vi "Normalize Score.vi"(10 "Value":dbl) -> (2 "Score":dbl)   [LabVIEW 2025]
doc: "Given a value with an ideal value of 1.0, normalize and map to a score that ranges between 0 and 100."
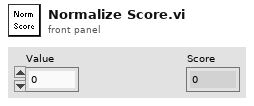
[diagram p1: front panel]
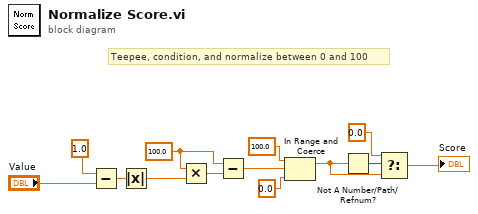
[diagram p0: block diagram]
diagram:
  w6 = 100.0 ("x/y")
  # "Teepee, condition, and normalize between 0 and 100"
  n1 = Subtract(x=1.0 ("y"), y="Value") -> (x-y=w8:dbl)
  n2 = Absolute Value(x=w8) -> (abs(x)=w5:dbl)
  n3 = Multiply(x=w6, y=w5) -> (x*y=w4:dbl)
  n4 = Subtract(x=w6, y=w4) -> (x-y=w9:dbl)
  n5 = In Range and Coerce(upper limit=100.0, x=w9, lower limit=0.0) -> (coerced(x)=w1:dbl)  [unwired: 1 out]
  n6 = Not A Number/Path/Refnum?(number/path/refnum=w1) -> (NaN/Path/Refnum?=w2:bool)
  n7 = Select(t=0.0 ("y"), s=w2, f=w1) -> (s? t:f=→"Score":dbl)
